vi "Destroy Data Channels.vi"(8 "error in":errorcluster, 11 "Node in":refnum<class "AMS Climate Chamber Template.lvclass">) -> (0 "error out":errorcluster, 3 "Node out":refnum<class "AMS Climate Chamber Template.lvclass">)   [LabVIEW 2023, in "AMS Climate Chamber Template.lvlib" / "AMS Climate Chamber Template.lvclass"]
uses:
  AMS Climate Chamber Template.lvclass
  AMS Climate Chamber Template.lvclass/AMS Climate Chamber Template.ctl
  C:/Program Files/National Instruments/AMS plugin/Capabilities/Capabilities/High Level Capabilities/Climate Chamber Cluster/Climate Chamber Cluster.lvclass
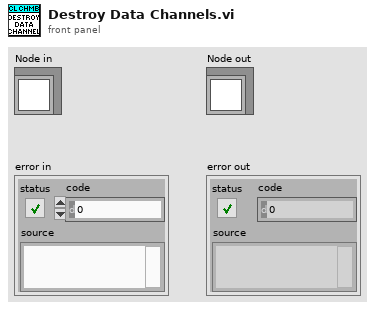
[diagram p1: front panel]
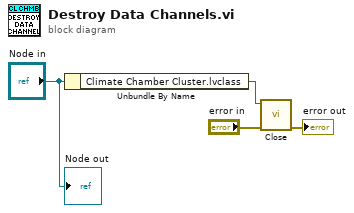
[diagram p0: block diagram]
diagram:
  n1 = Unbundle By Name("Node in") -> ("Climate Chamber Cluster.lvclass"=w3:refnum<class "Climate Chamber Cluster.lvclass">)
  n2 = call "Close.vi"("error in"="error in", "Climate Chamber Cluster.lvclass"=w3) -> ("error out"=→"error out":errorcluster)  [unwired: 9 in]
  "Node out" <- "Node in"
